vi "MuC_Read_DC.vi"(3 "error in (no error)":errorcluster, 4 "Delay / ms":u32, 5 "VISA resource name":refnum<visa-resource-name>) -> (0 "error out":errorcluster, 1 "Cmd":string, 2 "VISA resource name 2":refnum<visa-resource-name>)   [LabVIEW 2018]
doc: "Send a command to a MicroController telling it to read the data in buffer. \n\nIn the case of an DC read the microcontroller performs multiple reads and returns the largest value\n\nThe command for DC read as understood by the microcontroller is 'l' (for léigh or lis or leer or lesen etc)\n\nR. Sheehan 25 - 11 - 2020"
uses:
  <vilib>/regexp/Match Regular Expression.xnode
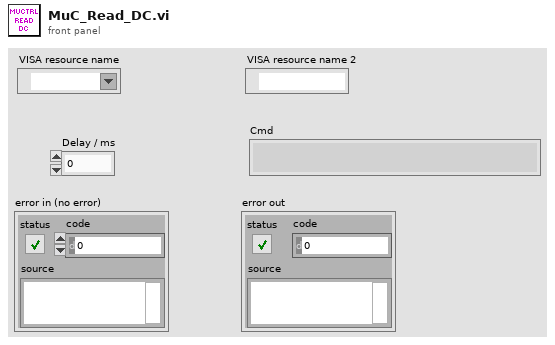
[diagram p1: front panel]
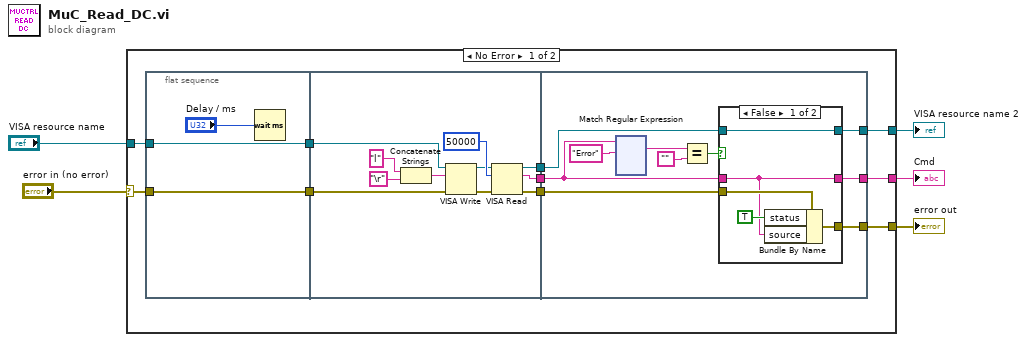
[diagram p0: block diagram]
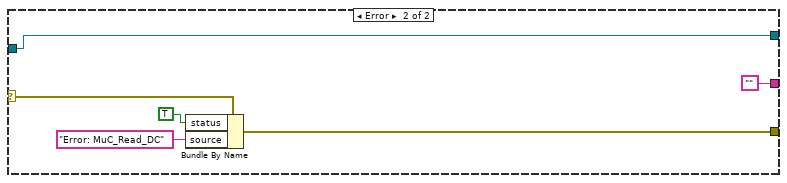
[diagram p3: hidden frame]
diagram:
  n1 = case shown="No Error" "error in (no error)" {
    selector: "error in (no error)" -> [w14 w167]
    tunnel: [w10 w166] -> w4
    tunnel: "VISA resource name" -> [w15 w163]
    tunnel: [w8 w163] -> w2
    tunnel: [w12 ""] -> w1
    frame No Error {
      n2 = flat-sequence {
        tunnel: w14 -> [w17]
        tunnel: w15 -> [w18]
        tunnel: [w18] -> w7
        tunnel: [w17] -> w6
        tunnel: [w21] -> w13
        tunnel: [w20] -> w11
        tunnel: [w19] -> w9
        tunnel: w7 -> [w23]
        tunnel: w6 -> [w22]
        tunnel: w13 -> [w35]
        tunnel: [w34] -> w12
        tunnel: w11 -> [w33]
        tunnel: [w32] -> w10
        tunnel: w9 -> [w31]
        tunnel: [w30] -> w8
        frame #0 {
          n3 = Wait (ms)(milliseconds to wait="Delay / ms") -> ()  [unwired: 1 out]
        }
        frame #1 {
          n4 = Concatenate Strings("l" ("string"), "\r") -> (w24:string)
          n5 = VISA Write(VISA resource name=w23, write buffer=w24, error in (no error)=w22) -> (VISA resource name out=w25:refnum<visa-resource-name>, error out=w26:errorcluster)  [unwired: 1 out]
          n6 = VISA Read(VISA resource name=w25, byte count=u32 50000, error in (no error)=w26) -> (VISA resource name out=w19:refnum<visa-resource-name>, read buffer=w21:string, error out=w20:errorcluster)  [unwired: 1 out]
        }
        frame #2 {
          n7 = xnode "Match Regular Expression"("input string"=w35, "regular expression"="Error") -> ("whole match"=w37:string)  [unwired: 4 in, 4 out]
          n8 = Equal?(x=w37, y="") -> (x = y?=w36:bool)
          n9 = case shown="False" w36 {
            tunnel: w35 -> [w41 w47]
            tunnel: [w41 w47] -> w34
            tunnel: w33 -> [w44 w46]
            tunnel: [w42 w46] -> w32
            tunnel: w31 -> [w40 w45]
            tunnel: [w40 w45] -> w30
            frame False {
              n10 = Bundle By Name(cluster=w44, "status"=TRUE, "source"=w41) -> (w42:errorcluster)
            }
            frame True {
            }
          }
        }
      }
    }
    frame Error {
      n11 = Bundle By Name(cluster=w167, "status"=TRUE, "source"="Error: MuC_Read_DC") -> (w166:errorcluster)
    }
  }
  "error out" <- w4
  "VISA resource name 2" <- w2
  "Cmd" <- w1
